vi "ShooterSpeedRegulateV2.vi"(0 "Shooter Speed":T1(ring)) -> (4 "ALL GOOD":bool, 10 "Motor 1 Output":dbl)   [LabVIEW 2012]
uses:
  Robot Global Data.vi
  Max'sToolKit/ConvertVoltageToPercentVbs.vi
  <vilib>/addons/control/pid/NI_PID_pid.lvlib
  <vilib>/addons/control/pid/pid.llb/PID (DBL).vi
panel:
  in  "Reset Shooter PID":bool
  out "Loop Rate (Hz)":dbl
  out "Array Index":dbl
  out "Wheel 1 RPS":dbl
  out "W1 Target RPS":dbl
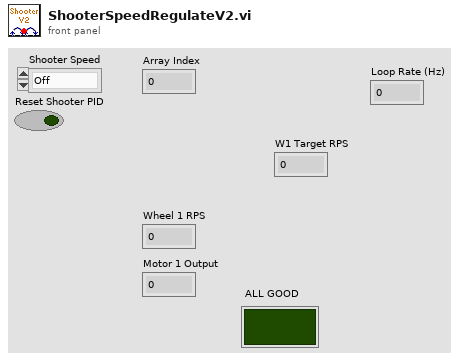
[diagram p1: front panel]
types:
  T1 = enum16{"Off", "Close Pyramid 3pt", "Far Pyramid 3pt", "Feeder Shot"}
  T2 = typedef "WPI_EncoderDevRef.ctl" = cluster{"DevStatus":errorcluster, "EncoderIndex":T3, "CounterIndex":T4, "DistancePerCount":dbl, "Decoding Type":T5}
  T3 = typedef "FPGA_EncoderIdx.ctl" = enum8{"Enc 0", "Enc 1", "Enc 2", "Enc 3", "Invalid"}
  T4 = typedef "FPGA_CounterCtrSystemIndex.ctl" = enum8{"Ctr 0", "Ctr 1", "Ctr 2", "Ctr 3", "Ctr 4", "Ctr 5", "Ctr 6", "Ctr 7", "Invalid"}
  T5 = typedef "WPI_EncoderType.ctl" = enum16{"1x", "2x", "4x"}
  T6 = cluster{"proportional gain (Kc)":dbl, "integral time (Ti, min)":dbl, "derivative time (Td, min)":dbl}
  T7 = typedef "WPI_MotorControlDeviceRef.ctl" = cluster{"DeviceStatus":errorcluster, "Type":enum16{"PWM", "CAN"}, "PWM":cluster{"Digital Module":T8, "PWM Channel":T9, "DeadBand":T10}, "CAN":cluster{"Device Number":u8, "Control Mode":T11, "Semaphore":T12, "Max Vout":dbl}, "Invert":bool, "TransformRef":T13, "InvTransformRef":T13}
  T8 = typedef "FPGA_TypedefDigitalModule.ctl" = enum16{"Digital Module 1", "Digital Module 2"}
  T9 = typedef "FPGA_DIOPWMChannel.ctl" = enum8{"PWM 1", "PWM 2", "PWM 3", "PWM 4", "PWM 5", "PWM 6", "PWM 7", "PWM 8", "PWM 9", "PWM 10", "Invalid"}
  T10 = typedef "WPI_PWMDeadband.ctl" = cluster{"Name":string, "maxPositivePwm":i32, "minPositivePwm":i32, "centerPwm":i32, "maxNegativePwm":i32, "minNegativePwm":i32, "angularRange":u16}
  T11 = typedef "WPI_CANJaguar_ControlMode.ctl" = enum8{"Percent VBus", "Current", "Speed", "Position", "Voltage"}
  T12 = typedef "Semaphore RefNum" = refnum<k1>
  T13 = typedef "WPI_PWMTransform_ConPane.ctl" = refnum<vi>
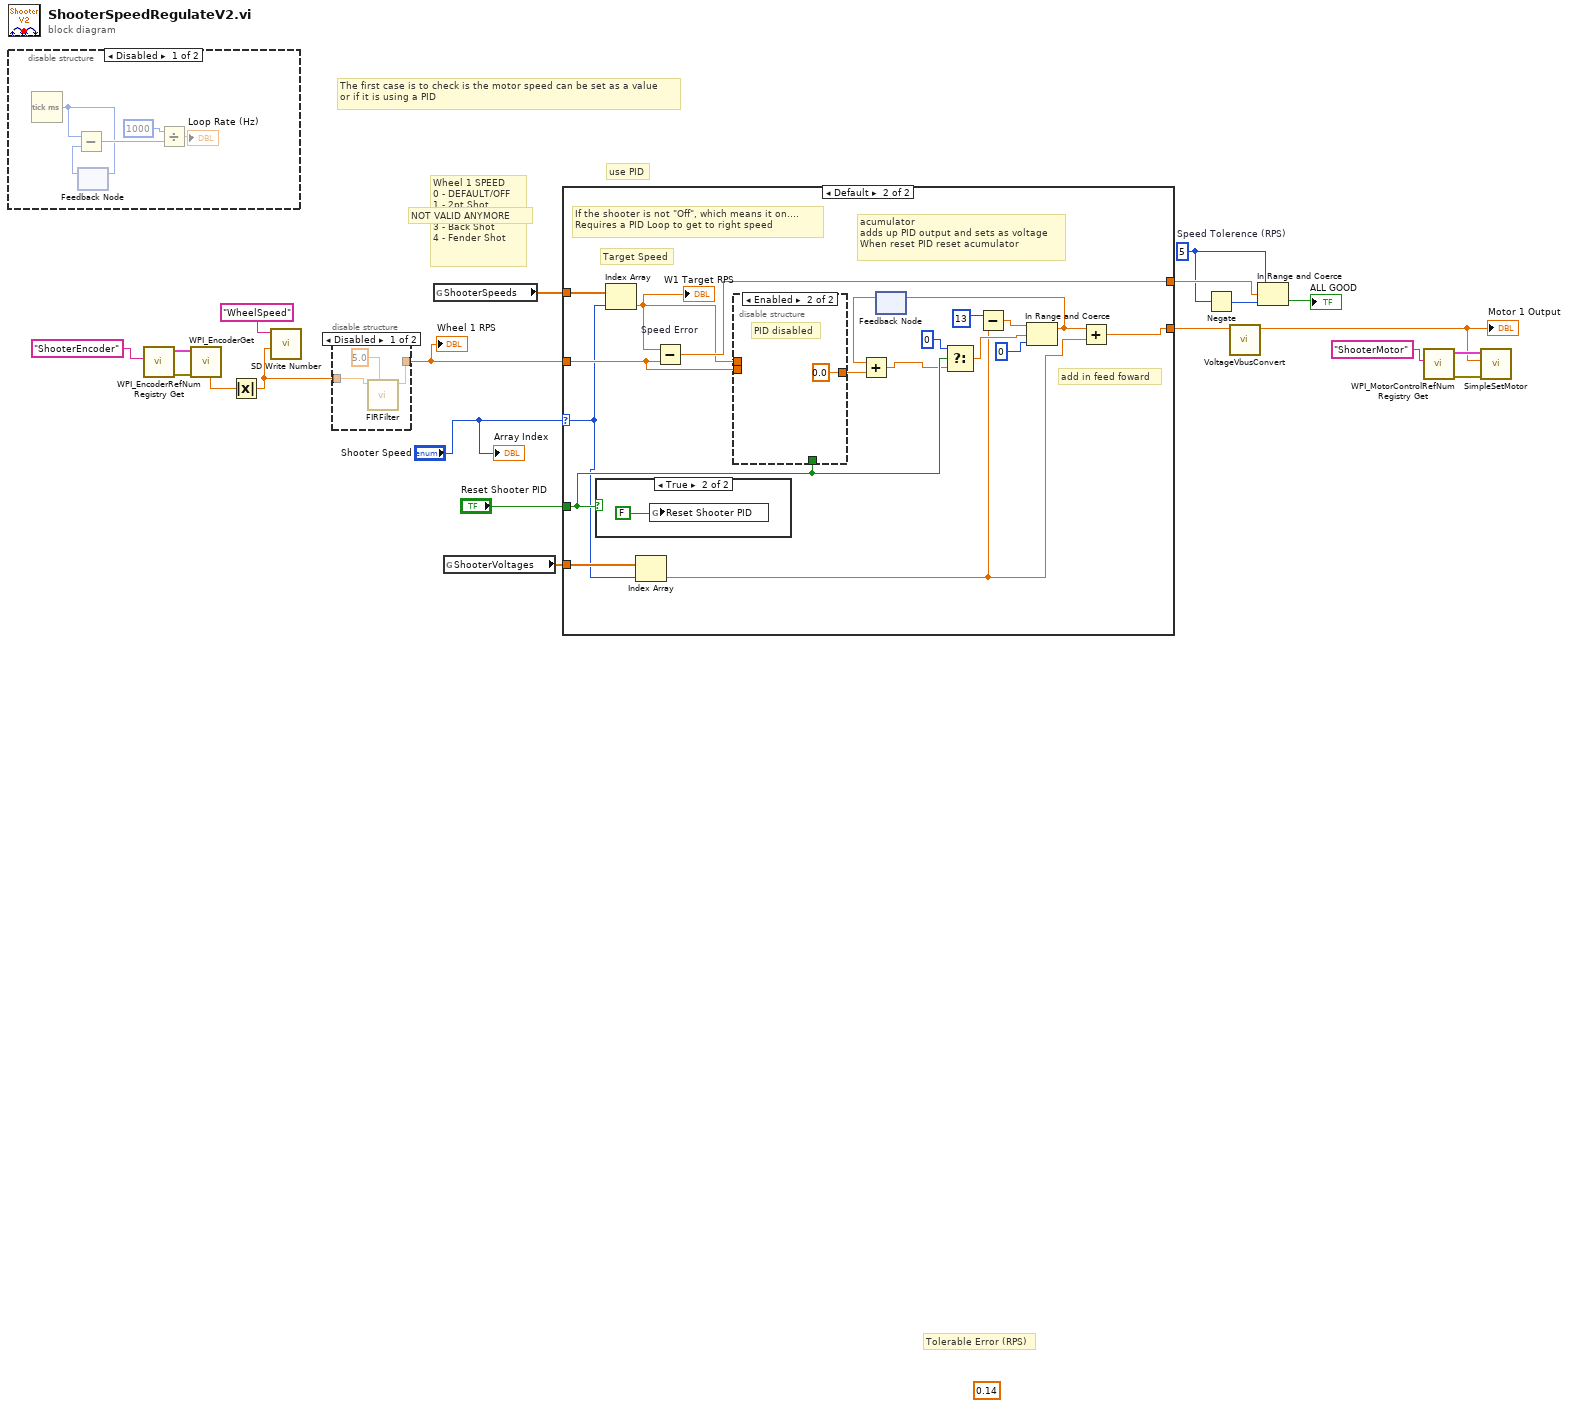
[diagram p0: block diagram]
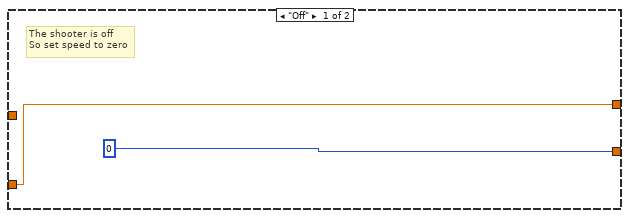
[diagram p4: hidden frame]
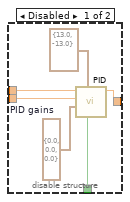
[diagram p5: hidden frame]
diagram:
  w7 = 5  # Speed Tolerence (RPS)
  (unwired) 0.14
  # "use PID"
  # "NOT VALID ANYMORE"
  # "The first case is to check is the motor speed can be set as a value\nor if it is using a PID"
  # "Tolerable Error (RPS)"
  # "Wheel 1 SPEED\n0 - DEFAULT/OFF\n1 - 2pt Shot\n2 - 3pt Key Shot\n3 - Back Shot\n4 - Fender Shot"
  n1 = disable-structure shown="Disabled" {
    frame Disabled {
      n2 = Tick Count (ms)() -> (millisecond timer value=w21:u32)
      n3 = feedback #1() -> (w22:u32)  [unwired: 1 in]
      n4 = Subtract(x=w21, y=w22) -> (x-y=w24:u32)
      n5 = feedback-in #1(w21) -> ()
      n6 = Divide(x=1000, y=w24) -> (x/y=→"Loop Rate (Hz)":dbl)
    }
    frame Enabled {
    }
  }
  n7 = call <vilib>:"WPI_EncoderRefNum Registry Get.vi"("refnum name"="ShooterEncoder") -> ("error out"=w13:errorcluster, "EncoderDevRef"=w14:T2)  [unwired: 9 in]
  n8 = call <vilib>:"WPI_EncoderGet.vi"("error in (no error)"=w13, "EncoderDevRef"=w14) -> ("Rate"=w10:dbl)  [unwired: 4 in, 5 out]
  n9 = Absolute Value(x=w10) -> (abs(x)=w2:dbl)
  n10 = call <vilib>:"SD Write Number.vi"("Numeric"=w2, "Name"="WheelSpeed") -> ()  [unwired: 8 in, 2 out]
  n11 = disable-structure shown="Disabled" {
    disable-tunnel: [w27 w29] -> w12
    disable-tunnel: w2 -> [w26 w29]
    frame Disabled {
      n12 = call "FIRFilter.vi"("Filter Size"=5.0 ("Filter size"), "Input"=w26) -> ("Output"=w27:dbl)  [unwired: 9 in]
    }
    frame Enabled {
    }
  }
  "Wheel 1 RPS" <- w12
  n13 = global read "Robot Global Data.vi" "ShooterSpeeds"() -> (w11:dbl[])
  n14 = global read "Robot Global Data.vi" "ShooterVoltages"() -> (w4:dbl[])
  n15 = case shown="Default" "Shooter Speed" {
    selector: "Shooter Speed" -> [_ w39]
    tunnel: w12 -> [w30 w47]
    tunnel: [0 w36] -> w6
    tunnel: [w30 w48] -> w16
    tunnel: w11 -> [_ w45]
    tunnel: "Reset Shooter PID" -> [_ w42]
    tunnel: w4 -> [_ w40]
    frame "Off" {
      # "The shooter is off\nSo set speed to zero"
    }
    frame Default {
      # "add in feed foward"
      # "acumulator\nadds up PID output and sets as voltage\nWhen reset PID reset acumulator"
      # "Target Speed"
      # "If the shooter is not \"Off\", which means it on....\nRequires a PID Loop to get to right speed"
      n16 = case shown="True" w42 {
        frame False {
        }
        frame True {
          n17 = global write "Robot Global Data.vi" "Reset Shooter PID"(FALSE) -> ()
        }
      }
      n18 = Index Array(array=w45, index=w39) -> (element=w43:dbl)
      "W1 Target RPS" <- w43
      n19 = Index Array(array=w40, index=w39) -> (element=w33:dbl)
      n20 = Subtract "Speed Error"(x=w43, y=w47) -> (x-y=w48:dbl)
      n21 = disable-structure shown="Enabled" {
        disable-tunnel: w47 -> [w53 _]
        disable-tunnel: w43 -> [w52 _]
        disable-tunnel: w42 -> [w51 _]
        disable-tunnel: [w50 0.0 ("output")] -> w41
        frame Disabled {
          w54 = T6 {"proportional gain (Kc)"=0.0, "integral time (Ti, min)"=0.0, "derivative time (Td, min)"=0.0}  # PID gains
          n22 = call-poly <vilib>:"PID.vi"("reinitialize? (F)"=w51, "output range"=cluster{"output high":dbl, "output low":dbl} {"output high"=13.0, "output low"=-13.0}, "PID gains"=w54, "process variable"=w53, "setpoint"=w52) -> ("output"=w50:dbl)  [unwired: 5 in, 1 out]
        }
        frame Enabled {
          # "PID disabled"
        }
      }
      n23 = feedback #2() -> (w44:dbl)  [unwired: 1 in]
      n24 = Add(x=w44, y=w41) -> (x+y=w35:dbl)
      n25 = Select(t=0, s=w42, f=w35) -> (s? t:f=w38:dbl)
      n26 = Subtract(x=13 ("upper limit"), y=w33) -> (x-y=w32:dbl)
      n27 = In Range and Coerce(upper limit=w32, x=w38, lower limit=0 ("upper limit")) -> (coerced(x)=w37:dbl)  [unwired: 1 out]
      n28 = feedback-in #2(w37) -> ()
      n29 = Add(x=w37, y=w33) -> (x+y=w36:dbl)
    }
  }
  n30 = Negate(x=w7) -> (-x=w17:i32)
  n31 = call-poly "VoltageVbusConvert.vi"("Voltage"=w6) -> ("Vbus"=w5:dbl)  [unwired: 10 in]
  "Motor 1 Output" <- w5
  n32 = In Range and Coerce(upper limit=w7, x=w16, lower limit=w17) -> (In Range?=→"ALL GOOD":bool)  [unwired: 1 out]
  n33 = call <vilib>:"WPI_MotorControlRefNum Registry Get.vi"("refnum name"="ShooterMotor") -> ("error out"=w18:errorcluster, "MotorControlDevRef"=w19:T7)  [unwired: 9 in]
  n34 = call "SimpleSetMotor.vi"("error in (no error)"=w18, "Output"=w5, "MotorControlDevRef"=w19) -> ()  [unwired: 7 in, 2 out]
  "Array Index" <- "Shooter Speed"
